vi "LoopTime.vi"() -> (3 "LoopTime":u32)   [LabVIEW 2013]
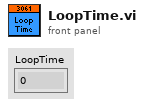
[diagram p1: front panel]
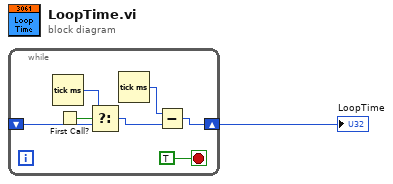
[diagram p0: block diagram]
diagram:
  n1 = while {
    shift-right: [w7] -> w1
    shift-left: _ -> [w4]
    stop <- TRUE stop-if-true
    n2 = Tick Count (ms)() -> (millisecond timer value=w3:u32)
    n3 = First Call?() -> (First Call?: T/F=w6:bool)
    n4 = Select(t=w3, s=w6, f=w4) -> (s? t:f=w5:u32)
    n5 = Tick Count (ms)() -> (millisecond timer value=w8:u32)
    n6 = Subtract(x=w8, y=w5) -> (x-y=w7:u32)
  }
  "LoopTime" <- w1
